vi "XYMetersToVoltageArray.vi"(8 "error in (no error)":errorcluster, 9 "Y Coordinate":dbl[](array[numeric]), 10 "X Coordinate":dbl[](array[numeric]), 11 "Asylum_Driver in":refnum<class "Asylum_Driver.lvclass">) -> (0 "error out":errorcluster, 1 "Y Voltage":dbl[](array[numeric]), 2 "X Voltage":dbl[](array[numeric]), 3 "Asylum_Driver out":refnum<class "Asylum_Driver.lvclass">)   [LabVIEW 2019, in "Asylum_Driver.lvclass"]
uses:
  Asylum_Driver.lvclass
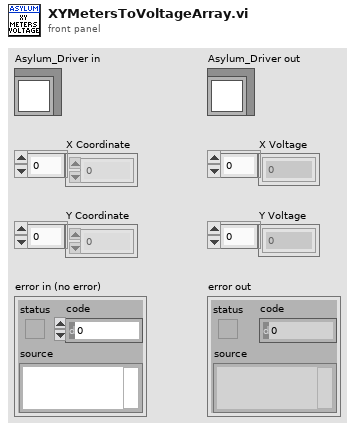
[diagram p1: front panel]
types:
  T1 = cluster{"XLVDT Sens":dbl, "YLVDT Sens":dbl, "XLVDT Offset":dbl, "YLVDT Offset":dbl}
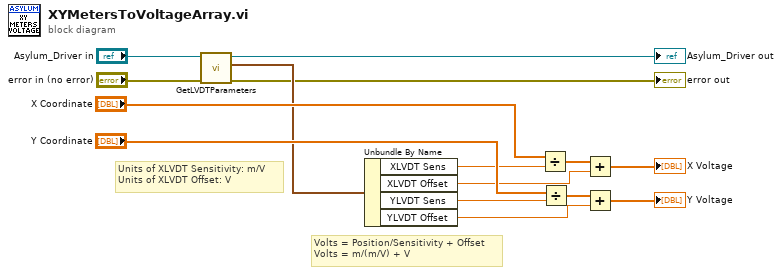
[diagram p0: block diagram]
diagram:
  # "Units of XLVDT Sensitivity: m/V\nUnits of XLVDT Offset: V"
  # "Volts = Position/Sensitivity + Offset\nVolts = m/(m/V) + V"
  n1 = call "GetLVDTParameters.vi"("error in (no error)"="error in (no error)", "Asylum_Driver in"="Asylum_Driver in") -> ("error out"=→"error out":errorcluster, "LVDT Parameters"=w5:T1, "Asylum_Driver out"=→"Asylum_Driver out":refnum<class "Asylum_Driver.lvclass">)  [unwired: 7 in]
  n2 = Unbundle By Name(w5) -> ("XLVDT Sens"=w6:dbl, "XLVDT Offset"=w8:dbl, "YLVDT Sens"=w7:dbl, "YLVDT Offset"=w11:dbl)
  n3 = Divide(x="X Coordinate", y=w6) -> (x/y=w9:dbl[])
  n4 = Divide(x="Y Coordinate", y=w7) -> (x/y=w10:dbl[])
  n5 = Add(x=w9, y=w8) -> (x+y=→"X Voltage":dbl[])
  n6 = Add(x=w10, y=w11) -> (x+y=→"Y Voltage":dbl[])
